vi "options.vi"(8 "Error In":errorcluster, 11 "QFontDialog In":refnum<class "QFontDialog.lvclass">) -> (0 "Error Out":errorcluster, 2 "Value":T1=1 items=["NoButtons"=1, "DontUseNativeDialog"=2, "ScalableFonts"=4, "NonScalableFonts"=8, "MonospacedFonts"=16, "ProportionalFonts"=32], 3 "QFontDialog Out":refnum<class "QFontDialog.lvclass">)   [LabVIEW 2014, in "QFontDialog.lvclass"]
doc: "LabVIEW-specific documentation is not yet available. See <b>http://doc.qt.io/qt-5/QFontDialog.html#options</b>"
uses:
  QFontDialog.lvclass
  FontDialogOption.ctl
  LQ Core/LQIdentity/LQIdentity.lvclass/LQIdentity.ctl
  LQ Core/LQ Core.lvlib
  LQ Core/LQIdentity/LQIdentity.lvclass
panel:
  # "Copyright (c) 2016 Sze Howe Koh\n\nThis Source Code Form is subject to the terms of the Mozilla Public\nLicense, v. 2.0. If a copy of the MPL was not distributed with this\nfile, You can obtain one at http://mozilla.org/MPL/2.0/."
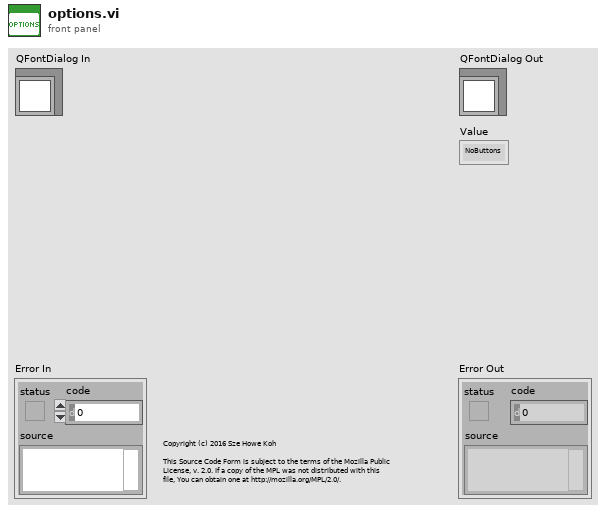
[diagram p1: front panel]
types:
  T1 = typedef "QFontDialog.lvclass/FontDialogOption.ctl" = i32
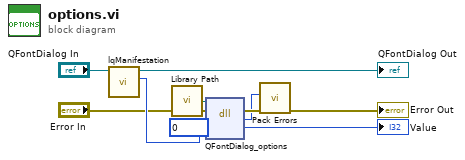
[diagram p0: block diagram]
diagram:
  w7 = T1 0 items=["NoButtons"=1, "DontUseNativeDialog"=2, "ScalableFonts"=4, "NonScalableFonts"=8, "MonospacedFonts"=16, "ProportionalFonts"=32] ("retVal")
  n1 = call "lqManifestation.vi"("LQIdentity in"="QFontDialog In") -> ("Manifestation"=w5:u64, "LQIdentity out"=→"QFontDialog Out":refnum<class "QFontDialog.lvclass">)  [unwired: 9 in]
  n2 = call "Library Path.vi"() -> ("Library Path"=w6:path)
  n3 = dll-call lib="?" fn="QFontDialog_options"(path in=w6, error in="Error In", "_retVal"=w7, "_instance"=w5) -> (error out=w3:errorcluster, w1:i32, "_retVal"=→"Value":i32)  [unwired: 2 in, 1 out]
  n4 = call "Pack Errors.vi"("Error In"=w3, "Error Code"=w1) -> ("Error Out"=→"Error Out":errorcluster)  [unwired: 9 in]
